vi "New VISA TCP Listener.vi"(8 "error in (no error)":errorcluster) -> (0 "error out":errorcluster, 3 "VISA TCP Listener out":refnum<class "VISA TCP Listener.lvclass">)   [LabVIEW 2021, in "Sockets.lvlib" / "VISA TCP Listener.lvclass"]
doc: "Constructor for a VISA TCP Listener.\nWebSockets 2.0.1.40\nSam Sharp - MediaMongrels Ltd\nCopyright (c) 2019, MediaMongrels Ltd"
uses:
  VISA TCP Listener.lvclass
  VISA TCP Listener.lvclass/VISA TCP Listener.ctl
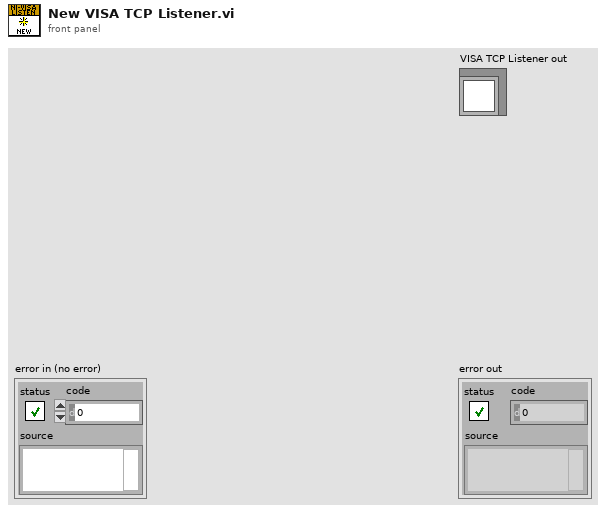
[diagram p1: front panel]
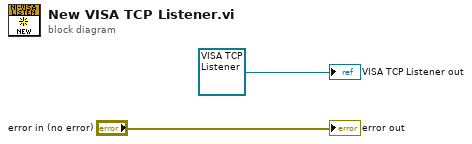
[diagram p0: block diagram]
diagram:
  "error out" <- "error in (no error)"
  "VISA TCP Listener out" <- refnum<class "VISA TCP Listener.lvclass"> refnum ("VISA TCP Listener in")
